vi "Load INI Config.vi"(8 "error in":errorcluster) -> (0 "error out":errorcluster)   [LabVIEW 2021]
uses:
  Controls/DAQ_Data.ctl
  Controls/Measure Type.ctl
  Controls/MUX_Data.ctl
  Controls/DMM_Data.ctl
  <vilib>/Utility/config.llb/Read Key (String).vi
  <vilib>/Utility/config.llb/NI_LVConfig.lvlib
panel:
  out "data":T1[](array[typedef])
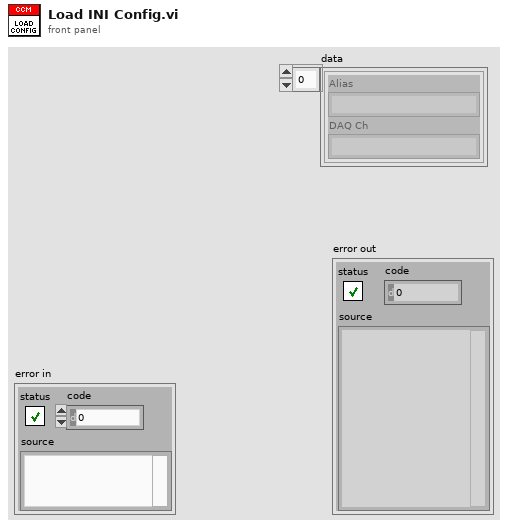
[diagram p1: front panel]
types:
  T1 = typedef "DAQ_Data.ctl" = cluster{"Alias":string, "DAQ Ch":string}
  T2 = typedef "NI_LVConfig.lvlib/Config Data RefNum.ctl" = refnum<k1>
  T3 = typedef "MUX_Data.ctl" = cluster{"Alias":string, "Topology":string}
  T4 = typedef "DMM_Data.ctl" = cluster{"Alias":string, "MUX":string, "Route":string}
  T5 = typedef "Measure Type.ctl" = enum16{"Analog_In", "Analog_Out", "Digital_In", "Digital_Out", "Switch", "NI_DMM"}
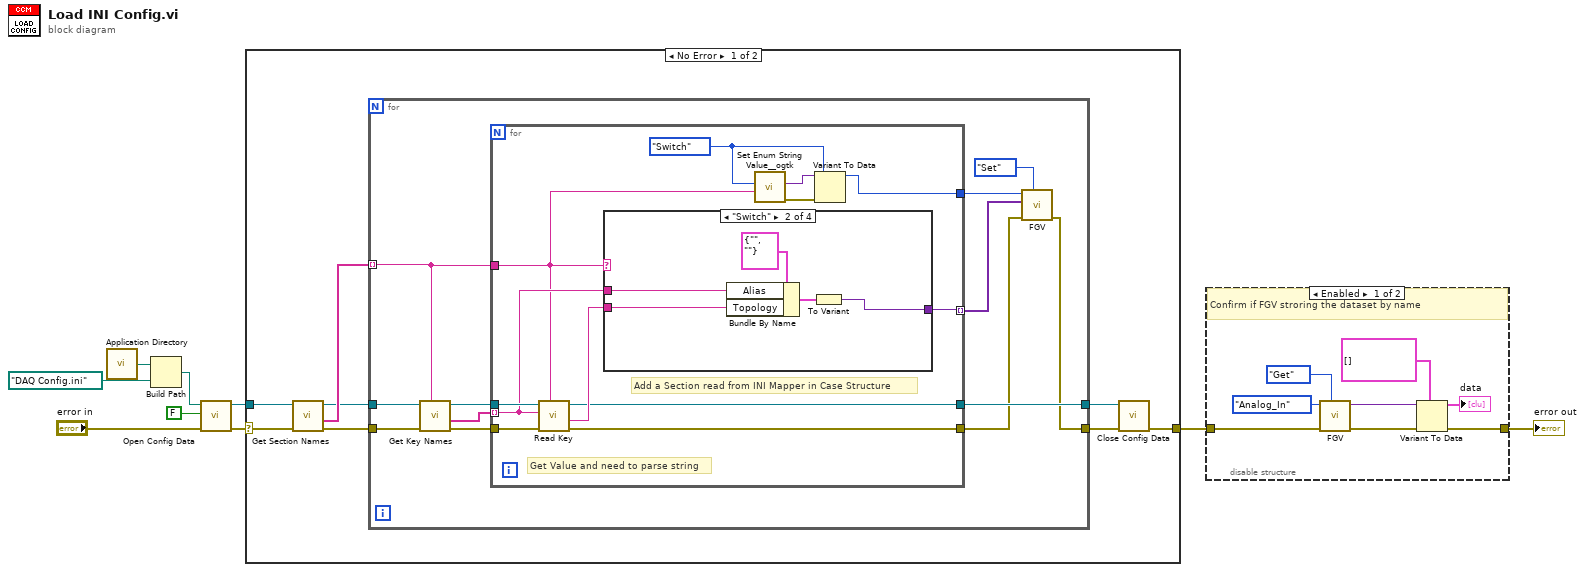
[diagram p0: block diagram]
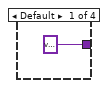
[diagram p2: hidden frame]
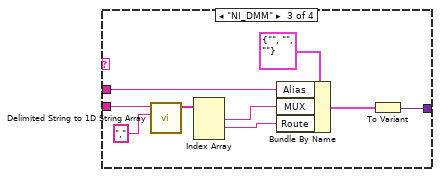
[diagram p3: hidden frame]
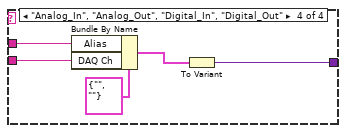
[diagram p4: hidden frame]
diagram:
  n1 = call <vilib>:"Application Directory.vi"() -> ("Application Directory"=w2:path)
  n2 = Build Path(base path=w2, name or relative path=path "DAQ Config.ini") -> (appended path=w1:path)
  n3 = call <vilib>:"Open Config Data.vi"("error in (no error)"="error in", "create file if necessary (T)"=FALSE, "configuration file path"=w1) -> ("error out"=w7:errorcluster, "refnum"=w8:T2)  [unwired: 6 in, 1 out]
  n4 = case shown="No Error" w7 {
    selector: w7 -> [w17 w62]
    tunnel: [w10 w62] -> w5
    tunnel: w8 -> [w16 _]
    frame No Error {
      n5 = call <vilib>:"Get Section Names.vi"("error in (no error)"=w17, "refnum"=w16) -> ("error out"=w14:errorcluster, "section names"=w15:string[], "refnum out"=w13:T2)  [unwired: 7 in]
      n6 = for {
        tunnel: w15 -> [w26] mode=indexing
        tunnel: w14 -> [w29]
        tunnel: w13 -> [w28]
        tunnel: [w27] -> w12
        tunnel: [w19] -> w11
        n7 = call <vilib>:"Get Key Names.vi"("section"=w26, "error in (no error)"=w29, "refnum"=w28) -> ("error out"=w25:errorcluster, "key names"=w24:string[], "refnum out"=w23:T2)  [unwired: 5 in, 1 out]
        n8 = for {
          tunnel: w25 -> [w41]
          tunnel: w24 -> [w38] mode=indexing
          tunnel: w26 -> [w32]
          tunnel: w23 -> [w40]
          tunnel: [w36] -> w27
          tunnel: [w39] -> w20
          tunnel: [w35] -> w21 mode=indexing
          tunnel: [w31] -> w18
          w30 = Measure_Type."Switch" ("Name")
          # "Add a Section read from INI Mapper in Case Structure"
          # "Get Value and need to parse string"
          n9 = call-poly <vilib>:"Read Key.vi"("section"=w32, "error in (no error)"=w41, "key"=w38, "refnum"=w40) -> ("error out"=w39:errorcluster, "value"=w37:string, "refnum out"=w36:T2)  [unwired: 4 in, 1 out]
          n10 = case shown="\"Switch\"" w32 {
            tunnel: w38 -> [_ w46 w50 w59]
            tunnel: w37 -> [_ w45 w53 w58]
            tunnel: [variant ("Variant") w44 w51 w61] -> w35
            frame Default {
            }
            frame "Switch" {
              n11 = Bundle By Name(cluster=T3 {"Alias"="", "Topology"=""}, "Alias"=w46, "Topology"=w45) -> (w43:T3)
              n12 = To Variant(anything=w43) -> (Variant=w44:variant)
            }
            frame "NI_DMM" {
              n13 = call <vilib>:"Delimited String to 1D String Array.vi"("delimiter"=",", "delimited string"=w53) -> ("string array"=w55:string[])  [unwired: 9 in]
              n14 = Index Array(array=w55) -> (element #1=w49:string, element #2=w48:string)  [unwired: 3 in, 1 out]
              n15 = Bundle By Name(cluster=T4 {"Alias"="", "MUX"="", "Route"=""} ("DAQ Data"), "Alias"=w50, "MUX"=w49, "Route"=w48) -> (w52:T4)
              n16 = To Variant(anything=w52) -> (Variant=w51:variant)
            }
            frame "Analog_In", "Analog_Out", "Digital_In", "Digital_Out" {
              n17 = Bundle By Name(cluster=T1 {"Alias"="", "DAQ Ch"=""} ("DAQ Data"), "Alias"=w59, "DAQ Ch"=w58) -> (w57:T1)
              n18 = To Variant(anything=w57) -> (Variant=w61:variant)
            }
          }
          n19 = call <userlib>:"Set Enum String Value__ogtk.vi"("String Value"=w32, "Default Enum Value"=w30) -> ("error out"=w34:errorcluster, "Enum"=w33:variant)  [unwired: 8 in]
          n20 = Variant To Data(error in=w34, type=w30, Variant=w33) -> (data=w31:T5)  [unwired: 1 out]
        }
        n21 = call "FGV.vi"("Method (Get)"=enum16{"Get", "Set"}."Set", "error in"=w20, "Data In"=w21, "Name"=w18) -> ("error out"=w19:errorcluster)  [unwired: 6 in, 1 out]
      }
      n22 = call <vilib>:"Close Config Data.vi"("error in (no error)"=w11, "refnum"=w12) -> ("error out"=w10:errorcluster)  [unwired: 8 in, 1 out]
    }
    frame Error {
    }
  }
  n23 = disable-structure shown="Enabled" {
    disable-tunnel: w5 -> [w70 w71]
    disable-tunnel: [w66 w71] -> w4
    frame Enabled {
      # "Confirm if FGV stroring the dataset by name"
      n24 = call "FGV.vi"("Method (Get)"=enum16{"Get", "Set"}."Get", "error in"=w70, "Name"=Measure_Type."Analog_In") -> ("error out"=w68:errorcluster, "Data out"=w67:variant)  [unwired: 7 in]
      n25 = Variant To Data(error in=w68, type=T1[] [], Variant=w67) -> (data=→"data":T1[], error out=w66:errorcluster)
    }
    frame Disabled {
    }
  }
  "error out" <- w4
